vi "Protocol Debug.vi"() -> ()   [LabVIEW 2025]
doc: "VI para hacer pruebas de funcionamiento de instrucciones y pines especificos\n(Este VI no deberia ser utilizable por estudiantes, solamente para pruebas, debugging o por docentes para explicar el funcionamiento de la trama de bytes)s"
panel:
  in  "stop":bool
  out "Comando enviado":string
  out "error out":errorcluster
  out "return count":u32
  out "Lectura":string
  in  "VISA resource name":refnum<visa-resource-name>
  in  "Instruccion":u8[](array[numeric]) format="%x"
  # "Ejemplo: Envío y recepción de datos por Serial (3 bytes)\nEste ejemplo muestra cómo construir y enviar una instrucción de 3 bytes en formato hexadecimal mediante el puerto serial en LV_ESP32, y cómo recibir un byte de respuesta. Está diseñado para depuración avanzada o para desarrollar nuevos VIs siguiendo un protocolo específico.\nNota: Este ejemplo demuestra cómo funciona el protocolo y no se recomienda para usuarios sin experiencia, ya que un uso incorrecto podría generar errores o comportamientos inesperados."
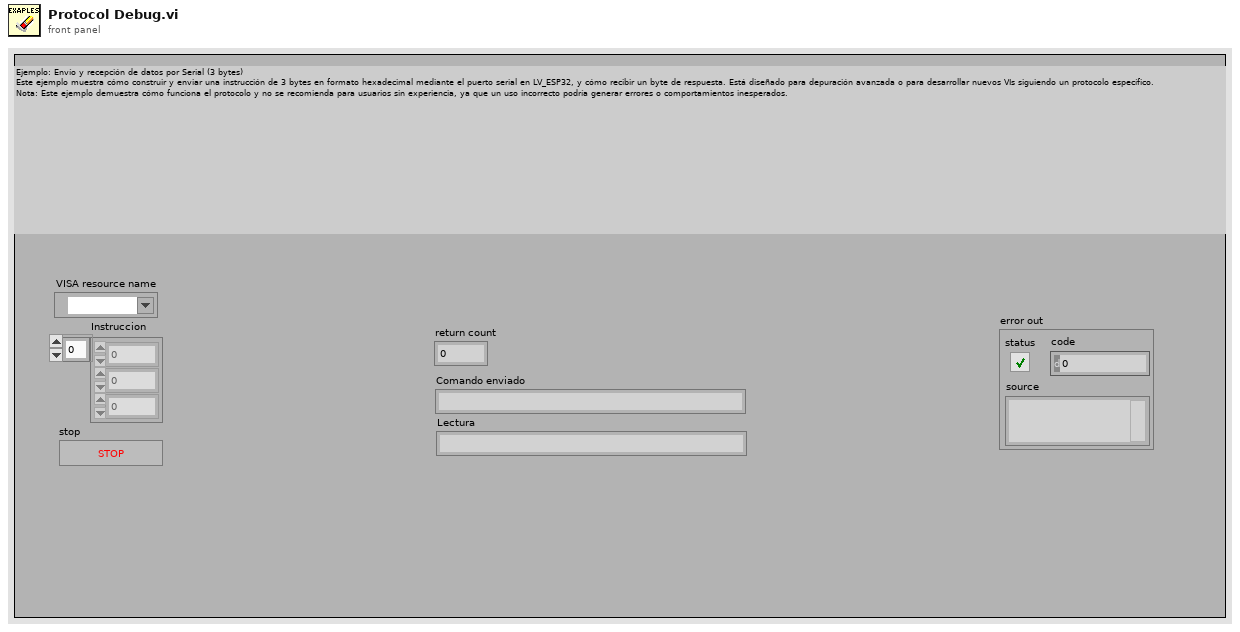
[diagram p1: front panel]
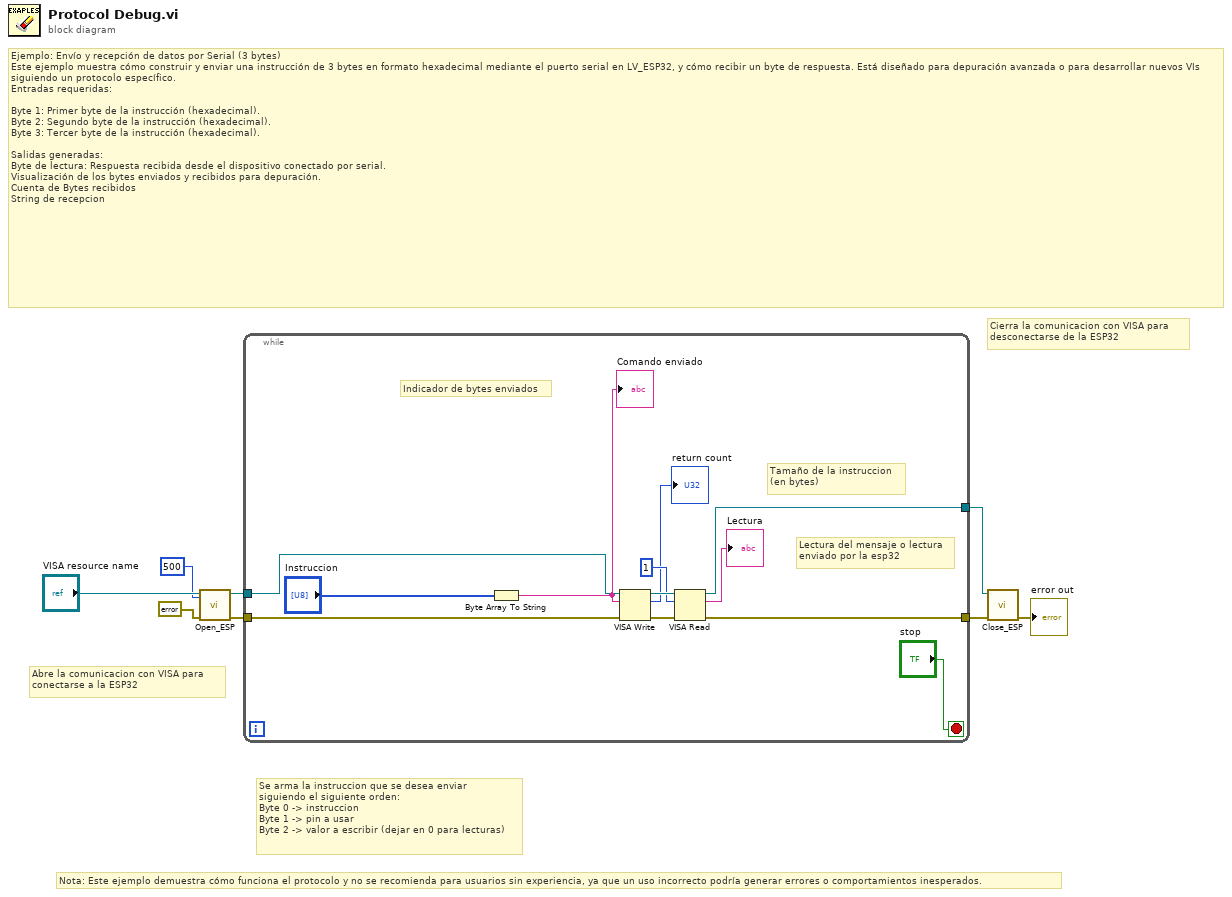
[diagram p0: block diagram]
diagram:
  # "Nota: Este ejemplo demuestra cómo funciona el protocolo y no se recomienda para usuarios sin experiencia, ya que un uso incorrecto podría generar errores o comportamientos inesperados."
  # "Ejemplo: Envío y recepción de datos por Serial (3 bytes)\nEste ejemplo muestra cómo construir y enviar una instrucción de 3 bytes en formato hexadecimal mediante el puerto serial en LV_ESP32, y cómo recibir un byte de respuesta. Está diseñado para depuración avanzada o para desarrollar nuevos VIs siguiendo un protocolo específico.\nEntradas requeridas:\n\nByte 1: Primer byte de la instrucción (hexadecimal).\nByte 2: Segundo byte de la instrucción (hexadecimal).\nByte 3: Tercer byte de la instrucción (hexadecimal).\n\nSalidas generadas:\nByte de lectura: Respuesta recibida desde el dispositivo conectado por serial.\nVisualización de los bytes enviados y recibidos para depuración.\nCuenta de Bytes recibidos\nString de recepcion"
  # "Cierra la comunicacion con VISA para\ndesconectarse de la ESP32"
  # "Abre la comunicacion con VISA para\nconectarse a la ESP32"
  # "Se arma la instruccion que se desea enviar\nsiguiendo el siguiente orden:\nByte 0 -> instruccion\nByte 1 -> pin a usar\nByte 2 -> valor a escribir (dejar en 0 para lecturas)"
  n1 = call "Open_ESP.vi"("timeout (10sec)"=u32 500, "error in (no error)"=errorcluster {"status"=FALSE, "code"=0, "source"=""}, "VISA resource name"="VISA resource name") -> ("error out"=w4:errorcluster, "VISA resource name out"=w8:refnum<visa-resource-name>)  [unwired: 7 in]
  n2 = while {
    tunnel: w8 -> [w18]
    tunnel: [w14] -> w3
    tunnel: w4 -> [w17]
    tunnel: [w13] -> w2
    stop <- "stop" stop-if-true
    # "Lectura del mensaje o lectura\nenviado por la esp32"
    # "Tamaño de la instruccion\n(en bytes)"
    # "Indicador de bytes enviados"
    n3 = Byte Array To String(unsigned byte array="Instruccion") -> (string=w19:string)
    "Comando enviado" <- w19
    n4 = VISA Write(VISA resource name=w18, write buffer=w19, error in (no error)=w17) -> (VISA resource name out=w15:refnum<visa-resource-name>, return count=→"return count":u32, error out=w16:errorcluster)
    n5 = VISA Read(VISA resource name=w15, byte count=u32 1, error in (no error)=w16) -> (VISA resource name out=w14:refnum<visa-resource-name>, read buffer=→"Lectura":string, error out=w13:errorcluster)  [unwired: 1 out]
  }
  n6 = call "Close_ESP.vi"("error in (no error)"=w2, "VISA resource name"=w3) -> ("error out"=→"error out":errorcluster)  [unwired: 9 in]
